vi "test1.vi"() -> ()   [LabVIEW 2019]
panel:
  out "Result":dbl
  in  "In  2":dbl
  in  "In 1":dbl
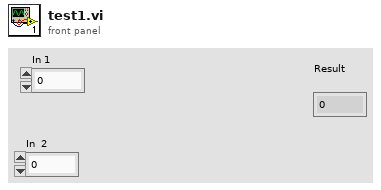
[diagram p1: front panel]
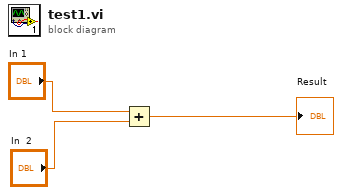
[diagram p0: block diagram]
diagram:
  n1 = Add(x="In 1", y="In  2") -> (x+y=→"Result":dbl)
